vi "Map_spectra2MapData.vi"(0 "Intensity":dbl[][](array[numeric]), 1 "Wavelength":dbl[](array[numeric]), 2 "XY Unique":cluster{"X Unique":dbl[], "Y Unique":dbl[]}, 5 "XY Full":cluster{dbl, dbl}[](array[cluster]), 6 "MapFunction":T1 items=["Total"=0, "Peak"=4, "Area"=2, "Value"=1, "Ratio"=3], 7 "X1":sgl, 9 "X2":sgl) -> (8 "MapZBounds":cluster{sgl, sgl}, 10 "MapData":sgl[][](array[numeric]))   [LabVIEW 2010]
uses:
  _TypeDefs/MapFunctions.ctl
panel:
  # "Runs all input spectra through the chosen evaluation method and generates a 2D array of result values to be inserted into an intensity graph."
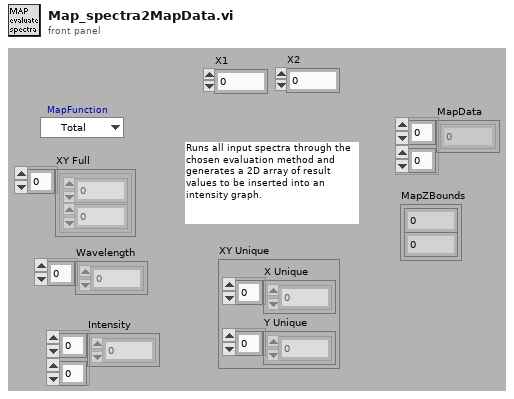
[diagram p1: front panel]
types:
  T1 = typedef "MapFunctions.ctl" = u16
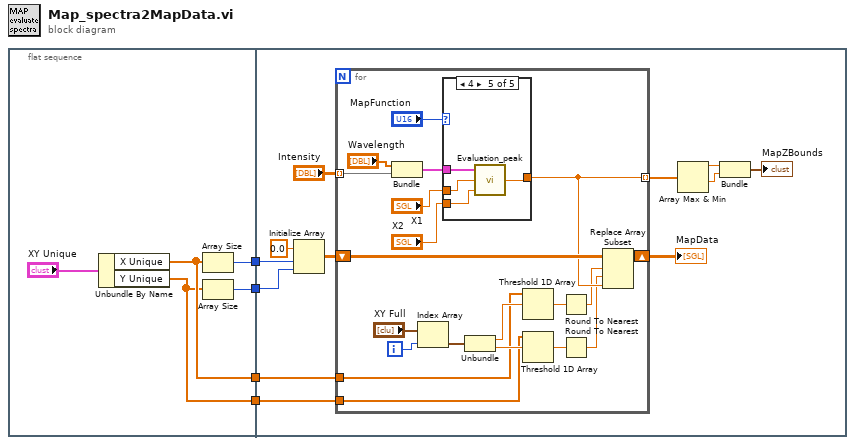
[diagram p0: block diagram]
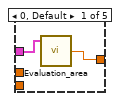
[diagram p2: hidden frame]
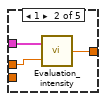
[diagram p3: hidden frame]
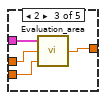
[diagram p4: hidden frame]
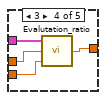
[diagram p5: hidden frame]
diagram:
  n1 = flat-sequence {
    tunnel: [w9] -> w4
    tunnel: [w8] -> w3
    tunnel: [w7] -> w2
    tunnel: [w6] -> w1
    tunnel: w4 -> [w12]
    tunnel: w3 -> [w13]
    tunnel: w2 -> [w11]
    tunnel: w1 -> [w10]
    frame #0 {
      n2 = Unbundle By Name("XY Unique") -> ("X Unique"=w7:dbl[], "Y Unique"=w6:dbl[])
      n3 = Array Size(array=w7) -> (size(s)=w9:i32)
      n4 = Array Size(array=w6) -> (size(s)=w8:i32)
    }
    frame #1 {
      n5 = Initialize Array(0.0 ("Element"), w12, w13) -> (w14:dbl[][])
      n6 = for {
        tunnel: "Intensity" -> [w37] mode=indexing
        tunnel: [w36] -> w20 mode=indexing
        shift-right: [w39] -> w17
        shift-left: w14 -> [w40]
        tunnel: w11 -> [w24]
        tunnel: w10 -> [w23]
        i -> [w25]
        n7 = Bundle("Wavelength"="Wavelength", "Intensity"=w37) -> (w41:cluster{"Wavelength":dbl[], "Intensity":dbl[]})  [unwired: 1 in]
        n8 = Index Array(array="XY Full", index=w25) -> (element=w28:cluster{dbl, dbl})
        n9 = case shown="4" "MapFunction" {
          tunnel: w41 -> [w43 w46 w50 w54 w58]
          tunnel: [w42 w45 w49 w53 w55] -> w36
          tunnel: "X1" -> [_ w44 w48 w52 w57]
          tunnel: "X2" -> [_ _ w47 w51 w56]
          frame 0, Default {
            n10 = call "Evaluation_area.vi"("Data"=w43) -> ("Area"=w42:sgl)  [unwired: 2 in]
          }
          frame 1 {
            n11 = call "Evaluation_intensity.vi"("X1"=w44, "DataXY"=w46) -> ("Y intensity"=w45:sgl)
          }
          frame 2 {
            n12 = call "Evaluation_area.vi"("X2"=w47, "X1"=w48, "Data"=w50) -> ("Area"=w49:sgl)
          }
          frame 3 {
            n13 = call "Evalutation_ratio.vi"("X2"=w51, "X1"=w52, "input cluster"=w54) -> ("PeaksRatio"=w53:sgl)
          }
          frame 4 {
            n14 = call "Evaluation_peak.vi"("X2"=w56, "X1"=w57, "Data"=w58) -> ("Area"=w55:sgl)
          }
        }
        n15 = Unbundle(w28) -> (w30:dbl, w31:dbl)
        n16 = Threshold 1D Array(2:w30, 3:w24) -> (0:w29:dbl)  [unwired: 1 in]
        n17 = Threshold 1D Array(2:w31, 3:w23) -> (0:w32:dbl)  [unwired: 1 in]
        n18 = Round To Nearest(number=w29) -> (nearest integer value=w27:dbl)
        n19 = Round To Nearest(number=w32) -> (nearest integer value=w26:dbl)
        n20 = Replace Array Subset(array=w40, new element=w36, index (row)=w27, index (col)=w26) -> (w39:dbl[][])
      }
      "MapData" <- w17
      n21 = Array Max & Min(array=w20) -> (max value=w18:sgl, min value=w19:sgl)  [unwired: 2 out]
      n22 = Bundle(w18, w19) -> (→"MapZBounds":cluster{sgl, sgl})  [unwired: 1 in]
    }
  }
